vi "setAngle.vi"(6 "Channel":i32, 8 "error in (no error)":errorcluster, 9 "Rate (°)/min)":dbl, 10 "Angle (°)":dbl, 11 "instrument.PPMS":refnum<class "instrument.PPMS.lvclass">) -> (0 "error out":errorcluster, 3 "instrument.PPMS out":refnum<class "instrument.PPMS.lvclass">)   [LabVIEW 2019, in "instrument.PPMS.lvclass"]
uses:
  instrument.PPMS.lvclass
  C:/Program Files (x86)/National Instruments/LabVIEW 2019/user.lib/LevyLab/Instrument Framework/Instrument/Instrument.lvclass
  <vilib>/AdvancedString/1D String Array to Delimited String.vi
  ff4c3b03-ec3b-4c30-b0c0-88201b2c7bd4.vi/8c4b539d-47e9-4523-a130-268f7a6aa968.vi
  <vilib>/Utility/Data Type/Get Type Information.vi
  <vilib>/Utility/Data Type/Get Numeric Information.vi
  <userlib>/_OpenG.lib/lvdata/lvdata.llb/Unwrap VVariant__ogtk.vi
  <userlib>/LevyLab/Instrument Framework/Instrument/API/Remote Client.vi
  <vilib>/Utility/error.llb/Error Cluster From Error Code.vi
  <userlib>/LevyLab/Instrument Framework/Instrument Types/Cryostat/Instrument.Cryostat.lvclass
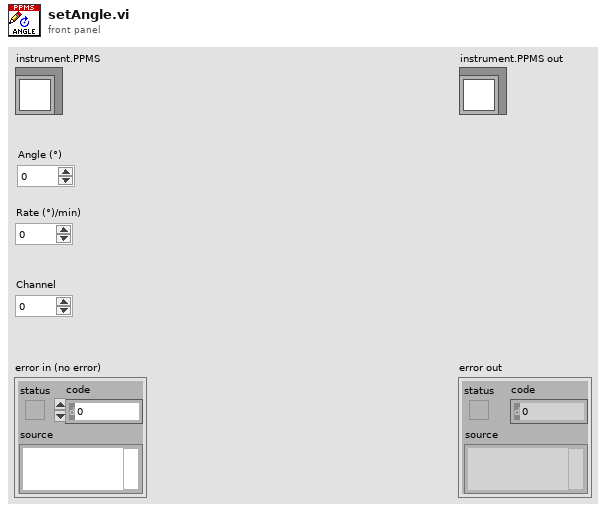
[diagram p1: front panel]
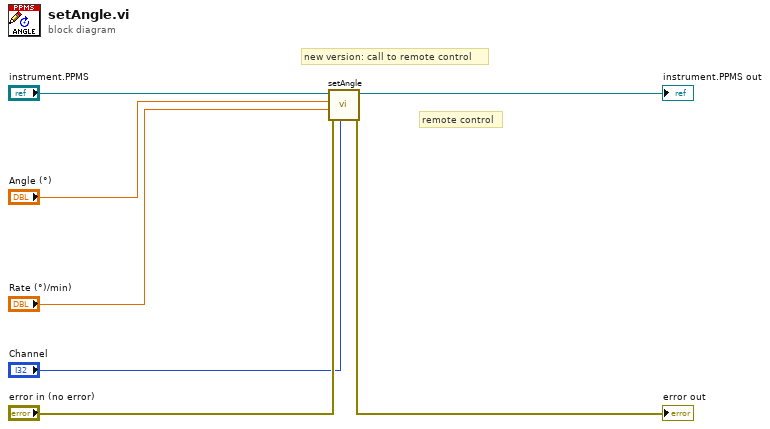
[diagram p0: block diagram]
diagram:
  # "remote control"
  # "new version: call to remote control"
  n1 = call-parent "setAngle.vi"("Channel"="Channel", "error in (no error)"="error in (no error)", "Rate (°/min)"="Rate (°)/min)", "Angle (°)"="Angle (°)", "Instrument.Cryostat in"="instrument.PPMS") -> ("error out"=→"error out":errorcluster, "Instrument.Cryostat out"=→"instrument.PPMS out":refnum<class "instrument.PPMS.lvclass">)  [unwired: 5 in]
